vi "Tegam4040 - Initialize.vi"(8 "error in (no error)":errorcluster, 9 "Reset? (T: Yes)":bool=TRUE, 11 "VISA Tegam4040":refnum<visa-resource-name>) -> (0 "error out":errorcluster, 3 "Instrument Session Handle":u32 format="%x")   [LabVIEW 2010, in "Tegam4040.lvlib"]
doc: "Establishes communication with the instrument and optionally performs an instrument reset. It also places the instrument in a default state needed for other instrument driver operations. Therefore, call this VI before calling other instrument driver VIs for this instrument. Generally, you need to call the <B>Initialize VI</B> only once at the beginning of an application."
uses:
  Tegam4040.lvlib
panel:
  # "© 2007 Tegam INC.  ALL RIGHTS RESERVED."
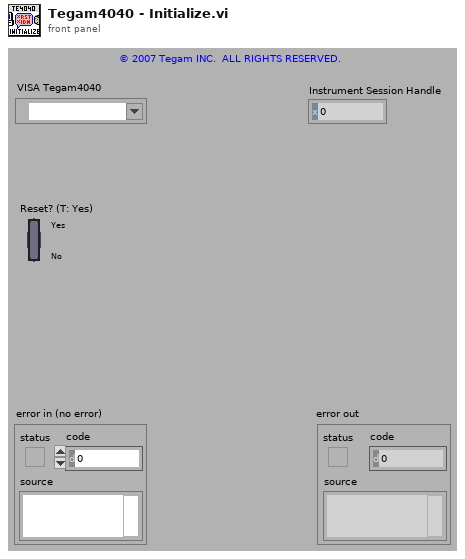
[diagram p1: front panel]
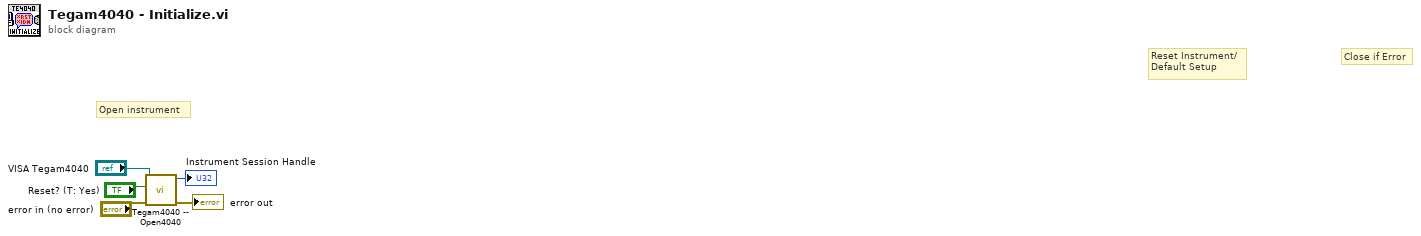
[diagram p0: block diagram]
diagram:
  # "Close if Error"
  # "Reset Instrument/\nDefault Setup"
  # "Open instrument"
  n1 = call "Tegam4040 -- Open4040.vi"("error in (no error)"="error in (no error)", "Reset Device?"="Reset? (T: Yes)", "VISA Resource In"="VISA Tegam4040") -> ("error out"=→"error out":errorcluster, "Instrument Session Handle"=→"Instrument Session Handle":u32)  [unwired: 7 in]
